vi "Launch Logger.vi"(8 "error in (no error)":errorcluster, 10 "Log Level":T2, 11 "Class Name":T1) -> (0 "error out":errorcluster)   [LabVIEW 2020, in "Logging.lvlib"]
uses:
  Logging.lvlib
  Define/Log Level.ctl
  Define/Log Option.ctl
  Global Log.vi
  Logger Mananger/Logger Mananger.lvclass
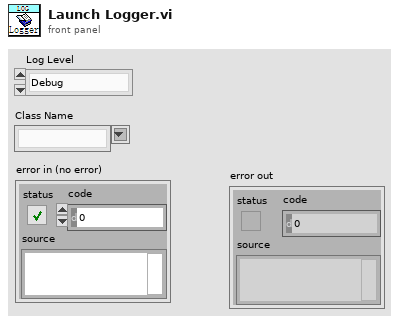
[diagram p1: front panel]
types:
  T1 = typedef "Logging.lvlib/Log Option.ctl" = string
  T2 = typedef "Logging.lvlib/Log Level.ctl" = enum16{"Debug", "Info", "Warn", "Error"}
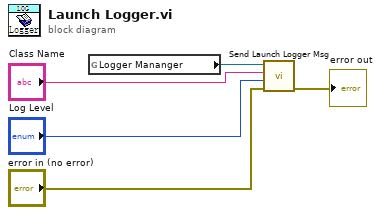
[diagram p0: block diagram]
diagram:
  n1 = global read "Global Log.vi" "Logger Mananger"() -> (w5:refnum<class "Logger Mananger.lvclass">)
  n2 = call "Send Launch Logger Msg.vi"("error in (no error)"="error in (no error)", "Log Level"="Log Level", "Logger Name"="Class Name", "Logger Mananger in"=w5) -> ("error out"=→"error out":errorcluster)  [unwired: 6 in, 1 out]
